vi "net方法-关闭模拟器.vi"   [LabVIEW 2017]
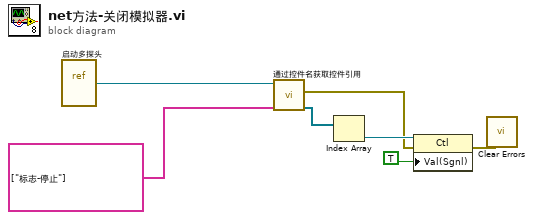
[diagram p0: block diagram]
diagram:
  n1 = vi-ref "启动多探头.vi"() -> (w7:refnum<vi>)
  n2 = call "通过控件名获取控件引用.vi"("控件名数组"=string[] ["标志-停止"], "VI引用"=w7) -> ("控件引用输出"=w5:refnum<vi>[], "错误输出"=w2:errorcluster)  [unwired: 7 in, 1 out]
  n3 = Index Array(array=w5) -> (element=w4:refnum<vi>)  [unwired: 1 in]
  n4 = property class="Ctl"(reference=w4, error in=w2, "Val(Sgnl)"=TRUE) -> (error out=w1:errorcluster)  [unwired: 1 out]
  n5 = call <vilib>:"Clear Errors.vi"("error in (no error)"=w1) -> ()  [unwired: 5 in, 2 out]
